vi "SPI Master with debug and stimulus [FPGA].vi"() -> ()   [LabVIEW 2011]
uses:
  <vilib>/Platform/TimedLoop/XDataNode/timing_clust.ctl
  <vilib>/Platform/TimedLoop/XDataNode/nitl_modes.ctl
  <vilib>/Platform/TimedLoop/XDataNode/wakeup.ctl
  SPI Master State.ctl
  <vilib>/rvi/interface/RandomDataEmulation/nirviRandomDataFPGAFIFO.vi
  <vilib>/rvi/interface/RandomDataEmulation/niFpgaRandomDataHandleErrors.vi
  <vilib>/Platform/TimedLoop/XDataNode/XDataNode.xnode
  <vilib>/rvi/DataTransferAndStorage/Container/XNode/niFpgaContainer.xnode
  <vilib>/rvi/interface/RandomDataEmulation/nirviRandomDataFpgaReadWriteTemplate.vi
  <vilib>/Platform/TimedLoop/XDataNode/XDNodeRunTimeDep.lvlib
panel:
  in  "Data Length":u8
  in  "HCP-1":u8
  out "Data Out":u32
  in  "Data In":u32
  in  "TX":bool
  in  "CPOL":bool
  in  "CPHA":bool
  in  "RESET":bool
  out "_SS":bool
  out "SCLK":bool
  out "MOSI":bool
  in  "MISO":bool
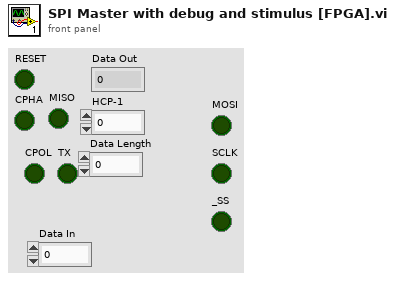
[diagram p1: front panel]
types:
  T1 = typedef "XDNodeRunTimeDep.lvlib/timing_clust.ctl" = cluster{"Expected End [f-1]":u64, "Actual End [f-1]":u64, "Finished Late? [f-1]":bool, "Expected End [i-1]":u64, "Actual End [i-1]":u64, "Finished Late? [i-1]":bool, "Expected Start [i]":u64, "Actual Start [i]":u64, "Expected Start [f]":u64, "Actual Start [f]":u64, "Source Name":string, "Structure Name":string, "Period":i64, "Deadline":i64, "Offset":i64, "Start":i64, "Priority":i32, "Timeout":i32, "Mode":T2, "Wakeup Reason":T3, "Error":errorcluster, "Source Type":string, "Secondary Source Type":string, "Global End Time":u64, "Global Start Time":u64, "Frame Duration":u64, "Iteration Duration":u64, "Assigned CPU":i32, "I/O Scan Engine Mode":u32}
  T2 = typedef "XDNodeRunTimeDep.lvlib/nitl_modes.ctl" = enum32{"No Change", "Process missed periods, maintain original phase", "Discard missed periods, maintain original phase", "Process missed periods, ignore original phase", "Discard missed periods, ignore original phase"}
  T3 = typedef "XDNodeRunTimeDep.lvlib/wakeup.ctl" = enum32{"Normal", "Aborted", "Asynchronous wakeup", "Timing source error", "Timed loop error", "Timeout"}
  T4 = typedef "SPI Master State.ctl" = enum8{"RESET", "Wait for TX", "Assert MOSI", "Toggle SCLK", "Latch MISO and Toggle SCLK", "Assert MOSI and Toggle SCLK"}
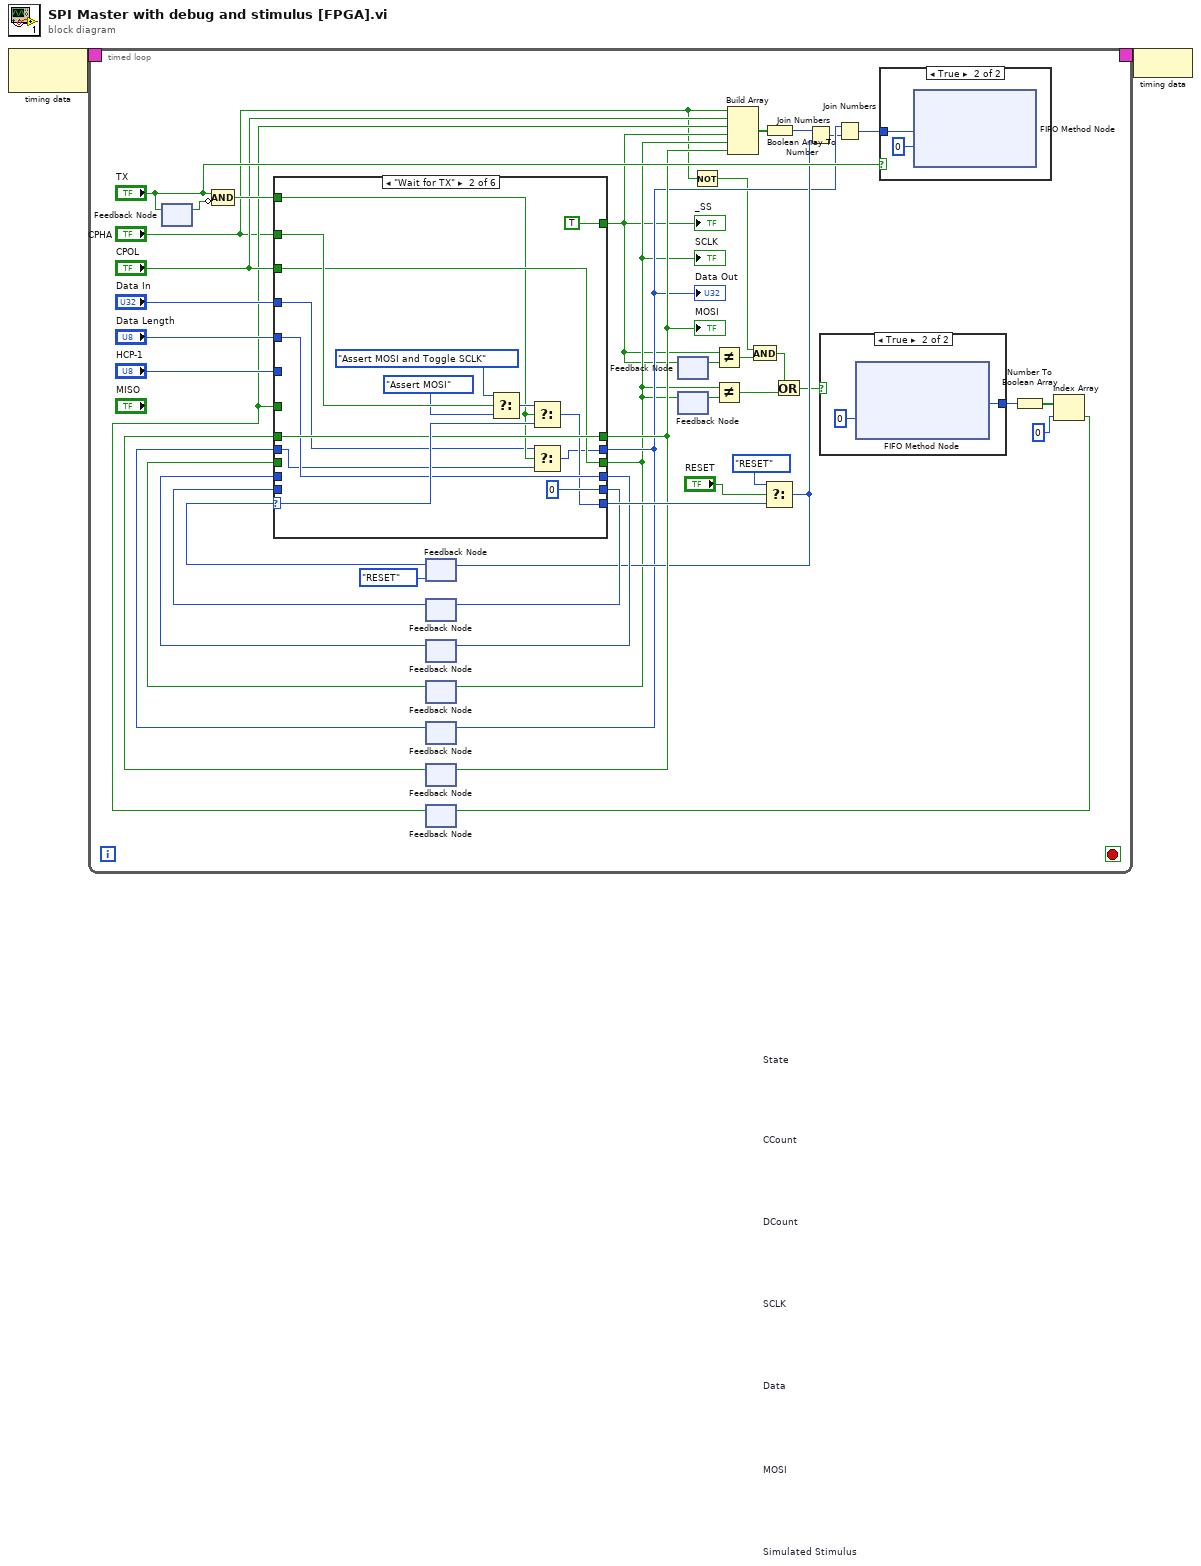
[diagram p0: block diagram]
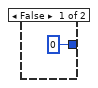
[diagram p2: hidden frame]
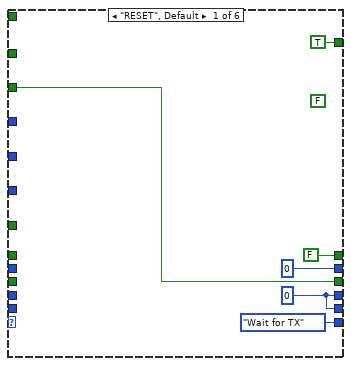
[diagram p4: hidden frame]
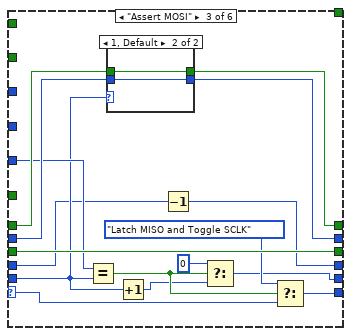
[diagram p5: hidden frame]
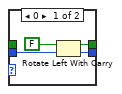
[diagram p6: hidden frame]
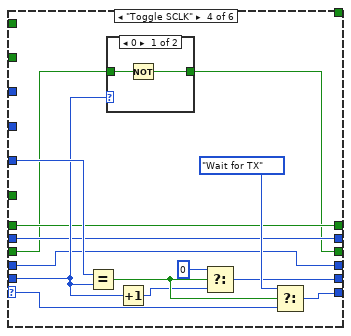
[diagram p7: hidden frame]
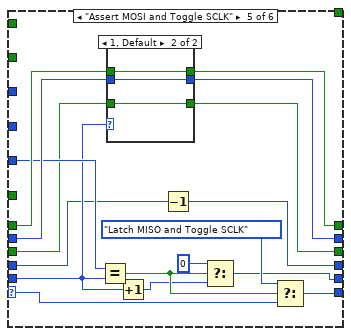
[diagram p9: hidden frame]
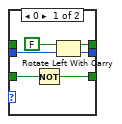
[diagram p10: hidden frame]
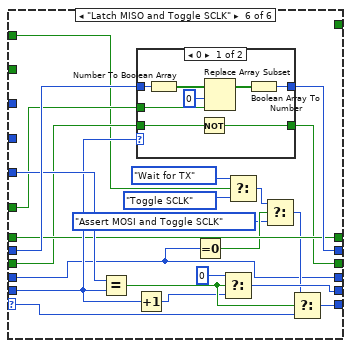
[diagram p11: hidden frame]
diagram:
  n1 = node-c288() -> (w2:T1)  [unwired: 1 in]
  n2 = timed-loop {
    timing: w2 -> [_]
    timing-out: [_] -> w1
    stop <- _ stop-if-true
    n3 = feedback #1() -> (w38:bool)  [unwired: 1 in]
    n4 = feedback-in #1("TX") -> ()
    n5 = Compound Arithmetic op=AND("TX", invert w38) -> (w30:bool)
    n6 = feedback #2 "State"(SPI_Master_State."RESET") -> (w42:T4)
    n7 = feedback #3 "CCount"() -> (w35:u8)  [unwired: 1 in]
    n8 = feedback #4 "DCount"() -> (w34:u8)  [unwired: 1 in]
    n9 = feedback #5 "SCLK"() -> (w33:bool)  [unwired: 1 in]
    n10 = feedback #6 "Data"() -> (w31:u32)  [unwired: 1 in]
    n11 = feedback #7 "MOSI"() -> (w29:bool)  [unwired: 1 in]
    n12 = feedback #8 "Simulated Stimulus"() -> (w11:bool)  [unwired: 1 in]
    n13 = case shown="\"Wait for TX\"" w42 {
      selector: w42 -> [_ w66 w78 w103 w119 w152]
      tunnel: [SPI_Master_State."Wait for TX" w59 w79 w104 w120 w153] -> w41
      tunnel: w30 -> [_ w58 _ _ _ _]
      tunnel: [w53 u8 0 w72 w97 w113 w147] -> w37
      tunnel: [w53 w61 w70 w96 w111 w135] -> w36
      tunnel: w35 -> [_ _ w75 w100 w116 w150]
      tunnel: w34 -> [_ _ w71 w96 w112 w135]
      tunnel: [TRUE ("MOSI") TRUE ("MOSI") _ _ _ _] -> w8
      tunnel: "CPHA" -> [_ w67 _ _ _ w141]
      tunnel: [w51 w60 w81 w92 w109 w143] -> w17
      tunnel: "CPOL" -> [w51 w60 _ _ _ _]
      tunnel: w33 -> [_ _ w81 w93 w110 w144]
      tunnel: "Data In" -> [_ w57 _ _ _ _]
      tunnel: [u32 0 ("Data In") w55 w84 w95 w124 w155] -> w19
      tunnel: w31 -> [_ w56 w85 w95 w125 w156]
      tunnel: "HCP-1" -> [_ _ w80 w105 w121 w154]
      tunnel: w11 -> [_ _ _ _ _ w145]
      tunnel: "Data Length" -> [_ w61 _ _ _ _]
      tunnel: [FALSE ("msb carry out") w62 w83 w94 w123 w146] -> w23
      tunnel: w29 -> [_ w62 w82 w94 w122 w146]
      frame "RESET", Default {
        (unwired) FALSE ("msb carry out")
        w53 = u8 0
      }
      frame "Wait for TX" {
        n14 = Select(t=SPI_Master_State."Assert MOSI and Toggle SCLK", s=w67, f=SPI_Master_State."Assert MOSI" ("t")) -> (s? t:f=w63:T4)
        n15 = Select(t=w63, s=w58, f=w66) -> (s? t:f=w59:T4)
        n16 = Select(t=w57, s=w58, f=w56) -> (s? t:f=w55:u32)
      }
      frame "Assert MOSI" {
        n17 = Equal?(x=w80, y=w75) -> (x = y?=w76:bool)
        n18 = case shown="1, Default" w75 {
          tunnel: w85 -> [w88 w90]
          tunnel: [w87 w90] -> w84
          tunnel: [w86 w91] -> w83
          tunnel: w82 -> [_ w91]
          frame 0 {
            n19 = Rotate Left With Carry(2:w88, 3:FALSE ("carry")) -> (0:w87:u32, 1:w86:bool)
          }
          frame 1, Default {
          }
        }
        n20 = Increment(x=w75) -> (x+1=w74:u8)
        n21 = Decrement(x=w71) -> (x-1=w70:u8)
        n22 = Select(t=u8 0, s=w76, f=w74) -> (s? t:f=w72:u8)
        n23 = Select(t=SPI_Master_State."Latch MISO and Toggle SCLK", s=w76, f=w78) -> (s? t:f=w79:T4)
      }
      frame "Toggle SCLK" {
        n24 = Equal?(x=w105, y=w100) -> (x = y?=w101:bool)
        n25 = case shown="0" w100 {
          tunnel: w93 -> [w107 w108]
          tunnel: [w106 w108] -> w92
          frame 0 {
            n26 = Not(x=w107) -> (.not. x?=w106:bool)
          }
          frame 1, Default {
          }
        }
        n27 = Increment(x=w100) -> (x+1=w99:u8)
        n28 = Select(t=u8 0, s=w101, f=w99) -> (s? t:f=w97:u8)
        n29 = Select(t=SPI_Master_State."Wait for TX", s=w101, f=w103) -> (s? t:f=w104:T4)
      }
      frame "Assert MOSI and Toggle SCLK" {
        n30 = Equal?(x=w121, y=w116) -> (x = y?=w117:bool)
        n31 = case shown="1, Default" w116 {
          tunnel: w125 -> [w130 w133]
          tunnel: [w129 w133] -> w124
          tunnel: [w128 w134] -> w123
          tunnel: w122 -> [_ w134]
          tunnel: w110 -> [w127 w132]
          tunnel: [w126 w132] -> w109
          frame 0 {
            n32 = Not(x=w127) -> (.not. x?=w126:bool)
            n33 = Rotate Left With Carry(2:w130, 3:FALSE ("carry")) -> (0:w129:u32, 1:w128:bool)
          }
          frame 1, Default {
          }
        }
        n34 = Increment(x=w116) -> (x+1=w115:u8)
        n35 = Decrement(x=w112) -> (x-1=w111:u8)
        n36 = Select(t=u8 0, s=w117, f=w115) -> (s? t:f=w113:u8)
        n37 = Select(t=SPI_Master_State."Latch MISO and Toggle SCLK", s=w117, f=w119) -> (s? t:f=w120:T4)
      }
      frame "Latch MISO and Toggle SCLK" {
        n38 = Equal?(x=w154, y=w150) -> (x = y?=w151:bool)
        n39 = Increment(x=w150) -> (x+1=w149:u8)
        n40 = case shown="0" w150 {
          tunnel: w156 -> [w164 w166]
          tunnel: [w159 w166] -> w155
          tunnel: w145 -> [w162 _]
          tunnel: w144 -> [w158 w165]
          tunnel: [w157 w165] -> w143
          frame 0 {
            n41 = Number To Boolean Array(number=w164) -> (Boolean array=w163:bool[])
            n42 = Not(x=w158) -> (.not. x?=w157:bool)
            n43 = Replace Array Subset(array=w163, new element=w162, index=0) -> (w160:bool[])
            n44 = Boolean Array To Number(Boolean array=w160) -> (number=w159:u32)
          }
          frame 1, Default {
          }
        }
        n45 = Equal To 0?(x=w135) -> (x = 0?=w142:bool)
        n46 = Select(t=u8 0, s=w151, f=w149) -> (s? t:f=w147:u8)
        n47 = Select(t=SPI_Master_State."Wait for TX", s=w141, f=SPI_Master_State."Toggle SCLK" ("t")) -> (s? t:f=w137:T4)
        n48 = Select(t=w137, s=w142, f=SPI_Master_State."Assert MOSI and Toggle SCLK" ("t")) -> (s? t:f=w139:T4)
        n49 = Select(t=w139, s=w151, f=w152) -> (s? t:f=w153:T4)
      }
    }
    "SCLK" <- w17
    "_SS" <- w8
    "MOSI" <- w23
    "Data Out" <- w19
    n50 = feedback-in #3(w37) -> ()
    n51 = feedback-in #4(w36) -> ()
    n52 = feedback-in #5(w17) -> ()
    n53 = feedback-in #6(w19) -> ()
    n54 = feedback-in #7(w23) -> ()
    n55 = feedback #9() -> (w10:bool)  [unwired: 1 in]
    n56 = feedback-in #9(w8) -> ()
    n57 = feedback #10() -> (w16:bool)  [unwired: 1 in]
    n58 = feedback-in #10(w17) -> ()
    n59 = Not(x="CPHA") -> (.not. x?=w3:bool)
    n60 = Not Equal?(x=w8, y=w10) -> (x != y?=w7:bool)
    n61 = Not Equal?(x=w17, y=w16) -> (x != y?=w9:bool)
    n62 = Build Array("CPHA", "CPOL", w11, w8, w17, w23) -> (w22:bool[])
    n63 = And(x=w3, y=w7) -> (x .and. y?=w6:bool)
    n64 = Select(t=SPI_Master_State."RESET", s="RESET", f=w41) -> (s? t:f=w21:T4)
    n65 = feedback-in #2(w21) -> ()
    n66 = Boolean Array To Number(Boolean array=w22) -> (number=w20:u8)
    n67 = Or(x=w6, y=w9) -> (x .or. y?=w5:bool)
    n68 = Join Numbers(hi=w20, lo=w21) -> ((hi.lo)=w18:u16)
    n69 = case shown="True" w5 {
      tunnel: [u64 0 ("Element") w45] -> w15
      frame False {
      }
      frame True {
        n70 = xnode ("FIFO Method Node")("Timeout"=0) -> ("Element"=w45:u64)  [unwired: 1 in, 2 out]
      }
    }
    n71 = Join Numbers(hi=w19, lo=w18) -> ((hi.lo)=w25:u64)
    n72 = case shown="True" "TX" {
      tunnel: w25 -> [_ w47]
      frame False {
      }
      frame True {
        n73 = xnode ("FIFO Method Node")("Element"=w47, "Timeout"=0) -> ()  [unwired: 1 in, 2 out]
      }
    }
    n74 = Number To Boolean Array(number=w15) -> (Boolean array=w14:bool[])
    n75 = Index Array(array=w14, index=0) -> (element=w12:bool)
    n76 = feedback-in #8(w12) -> ()
  }
  n77 = node-c288(w1) -> ()
